vi "connect.vi"(5 "output chunk queue size":u64=5000, 6 "timeout":i32, 7 "stream buffer size":u64=5242880, 8 "error in":errorcluster, 9 "port":string, 10 "host":string, 11 "client connector in":refnum<class "client connector.lvclass">) -> (0 "error out":errorcluster, 3 "connection out":refnum<class "connection.lvclass">)   [LabVIEW 2016, in "client connector.lvclass"]
uses:
  client connector.lvclass
  C:/Users/IEUser/Desktop/libasynclvtls/tls classes/connection creator/connection creator.lvclass
  connection/connection.lvclass
  connection creator.lvclass/connection creator.ctl
  dllwrapper/action complete event.ctl
  dllwrapper/async tls dl.lvlib
  connection creator.lvclass
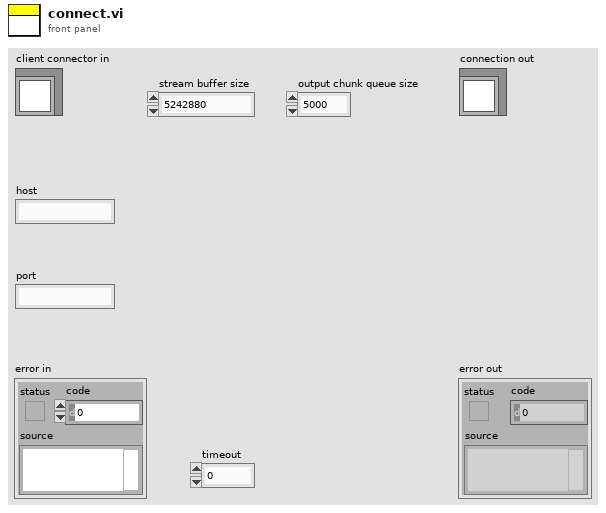
[diagram p1: front panel]
types:
  T1 = typedef "async tls dl.lvlib/action complete event.ctl" = cluster{"request ID":u32, "error code":i32, "error string":string}
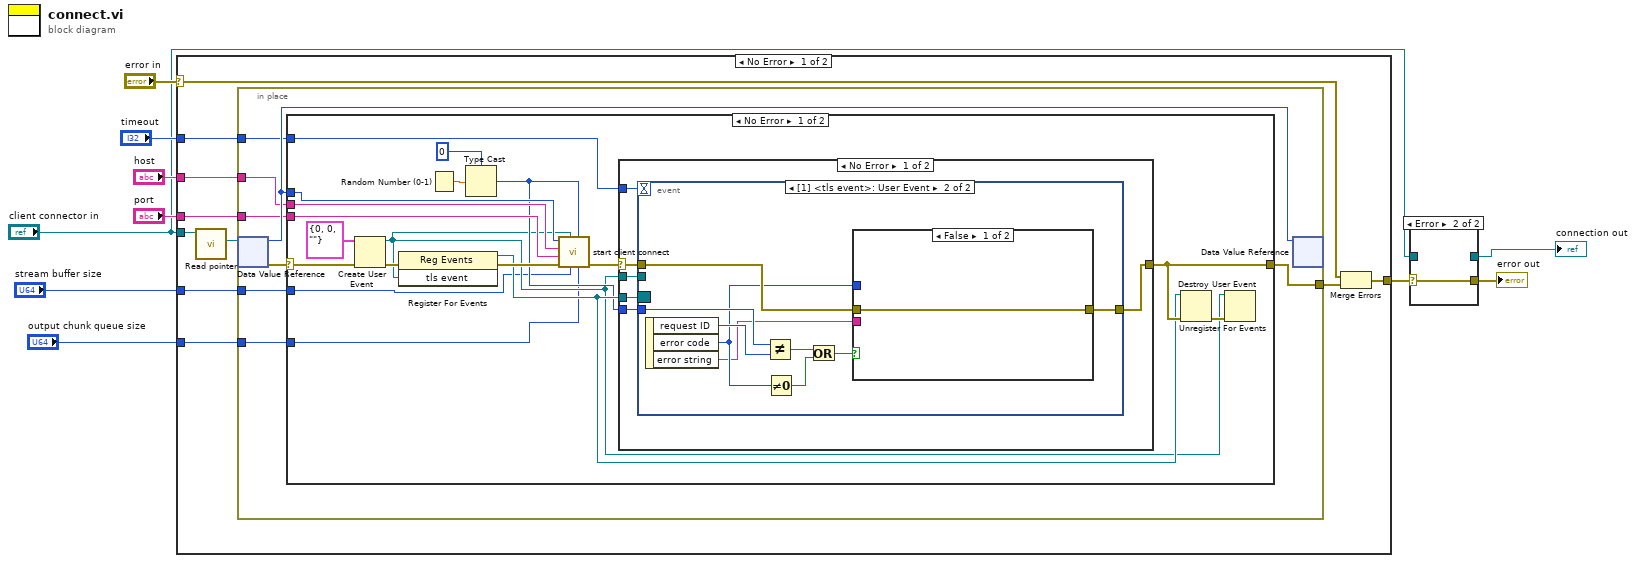
[diagram p0: block diagram]
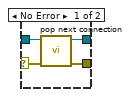
[diagram p2: hidden frame]
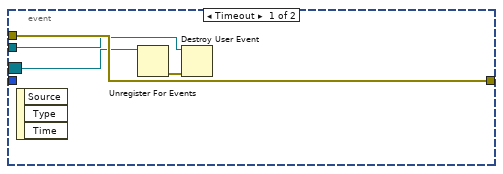
[diagram p3: hidden frame]
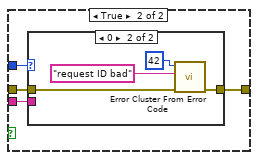
[diagram p4: hidden frame]
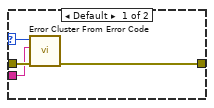
[diagram p5: hidden frame]
diagram:
  n1 = case shown="No Error" "error in" {
    selector: "error in" -> [w18 w81]
    tunnel: [w17 w81] -> w6
    tunnel: "client connector in" -> [w20 _]
    tunnel: "timeout" -> [w15 _]
    tunnel: "host" -> [w14 _]
    tunnel: "port" -> [w13 _]
    tunnel: "stream buffer size" -> [w12 _]
    tunnel: "output chunk queue size" -> [w11 _]
    frame No Error {
      n2 = call "Read pointer.vi"("connection creator in"=w20) -> ("pointer"=w19:refnum<data-value>)  [unwired: 10 in]
      n3 = in-place {
        in-place-border: [w27] -> w16
        in-place-border: w15 -> [w25]
        in-place-border: w14 -> [w24]
        in-place-border: w13 -> [w23]
        in-place-border: w12 -> [w22]
        in-place-border: w11 -> [w21]
        n4 = in-place-dvr #1(w19) -> (w26:u64, w28:errorcluster)
        n5 = case shown="No Error" w28 {
          selector: w28 -> [w43 w80]
          tunnel: [w42 w80] -> w27
          tunnel: w26 -> [w40 _]
          tunnel: w25 -> [w39 _]
          tunnel: w24 -> [w37 _]
          tunnel: w23 -> [w36 _]
          tunnel: w22 -> [w30 _]
          tunnel: w21 -> [w29 _]
          frame No Error {
            n6 = Create User Event(user event datatype=T1 {"request ID"=0, "error code"=0, "error string"=""} ("tls event"), error in=w43) -> (user event=w32:refnum<user-event>, error out=w46:errorcluster)
            n7 = register-events(error in=w46, w32) -> (reference out=w38:refnum<event-registration>, error out=w45:errorcluster)  [unwired: 1 in]
            n8 = Random Number (0-1)() -> (number: 0 to 1=w35:dbl)
            n9 = Type Cast(type=u32 0 ("request id"), x=w35) -> (*(type *) &x=w33:u32)
            n10 = call "start client connect.vi"("outQueueSize"=w29, "request id"=w33, "bufferMaxSize"=w30, "event"=w32, "error in"=w45, "port"=w36, "host"=w37, "client"=w40) -> ("error out"=w44:errorcluster)  [unwired: 3 in]
            n11 = case shown="No Error" w44 {
              selector: w44 -> [w49 w79]
              tunnel: [w48 w79] -> w42
              tunnel: w39 -> [w52 _]
              tunnel: w38 -> [w51 _]
              tunnel: w33 -> [w50 _]
              tunnel: w32 -> [w47 _]
              frame No Error {
                n12 = event shown="[1] <tls event>: User Event" {
                  selector: w51 -> [w55 _]
                  dyn-events: _ -> [_ _]
                  timeout: w52 -> [_ _]
                  tunnel: w50 -> [_ w65]
                  tunnel: w49 -> [w56 w60]
                  tunnel: [w56 w59] -> w48
                  tunnel: w47 -> [w53 _]
                  event Timeout {
                    n13 = event-data() -> ()  [unwired: 1 in, 3 out]
                    n14 = Unregister For Events(event registration refnum=w55) -> (error out=w54:errorcluster)  [unwired: 1 in]
                    n15 = Destroy User Event(user event=w53, error in=w54) -> ()  [unwired: 1 out]
                  }
                  event User Event {
                    n16 = event-data() -> ("request ID"=w63:u32, "error code"=w58:i32, "error string"=w57:string)  [unwired: 1 in]
                    n17 = Not Equal?(x=w65, y=w63) -> (x != y?=w64:bool)
                    n18 = Not Equal To 0?(x=w58) -> (x != 0?=w62:bool)
                    n19 = Or(x=w64, y=w62) -> (x .or. y?=w61:bool)
                    n20 = case shown="False" w61 {
                      tunnel: w60 -> [w66 w69]
                      tunnel: [w66 w70] -> w59
                      tunnel: w58 -> [_ w68]
                      tunnel: w57 -> [_ w67]
                      frame False {
                      }
                      frame True {
                        n21 = case shown="0" w68 {
                          selector: w68 -> [w72 _]
                          tunnel: [w74 w77] -> w70
                          tunnel: w69 -> [w73 w78]
                          tunnel: w67 -> [w71 _]
                          frame Default {
                            n22 = call <vilib>:"Error Cluster From Error Code.vi"("error in (no error)"=w73, "error message (\"\")"=w71, "error code (0)"=w72) -> ("error out"=w74:errorcluster)  [unwired: 6 in]
                          }
                          frame 0 {
                            n23 = call <vilib>:"Error Cluster From Error Code.vi"("error in (no error)"=w78, "error message (\"\")"="request ID bad" ("error message (\"\")"), "error code (0)"=42) -> ("error out"=w77:errorcluster)  [unwired: 6 in]
                          }
                        }
                      }
                    }
                  }
                }
              }
              frame Error {
              }
            }
            n24 = Unregister For Events(event registration refnum=w38, error in=w42) -> (error out=w41:errorcluster)
            n25 = Destroy User Event(user event=w32, error in=w41) -> ()  [unwired: 1 out]
          }
          frame Error {
          }
        }
        n26 = in-place-dvr #1(w26) -> ()  [unwired: 2 out]
      }
      n27 = Merge Errors(w18, w16) -> (w17:errorcluster)
    }
    frame Error {
    }
  }
  n28 = case shown="Error" w6 {
    selector: w6 -> [w85 w86]
    tunnel: [w84 w86] -> w5
    tunnel: "client connector in" -> [w83 _]
    tunnel: [w82 _] -> w3
    frame No Error {
      n29 = call "pop next connection.vi"("error in"=w85, "connection creator in"=w83) -> ("error out"=w84:errorcluster, "connection out"=w82:refnum<class "connection.lvclass">)  [unwired: 8 in]
    }
    frame Error {
    }
  }
  "error out" <- w5
  "connection out" <- w3
